vi "Get SMO RC Type.vi"(8 "error in (no error)":errorcluster, 11 "ExampleInstrument in":refnum<class "Instrument.Element2.lvclass">) -> (0 "error out":errorcluster, 2 "Configuration.SMO.RC Type":T1=enum."STM", 3 "ExampleInstrument out":refnum<class "Instrument.Element2.lvclass">)   [LabVIEW 2019, in "Instrument.Element2.lvclass"]
uses:
  Instrument.Element2.lvclass
  <userlib>/LevyLab/Instrument Framework/SMOs/RemoteControl/Typedefs/RC Com Type--enum.ctl
  <userlib>/LevyLab/Instrument Framework/Instrument Types/VSource/Instrument.VSource.lvclass
  <userlib>/LevyLab/Instrument Framework/SMOs/RemoteControl/RemoteControl.lvclass
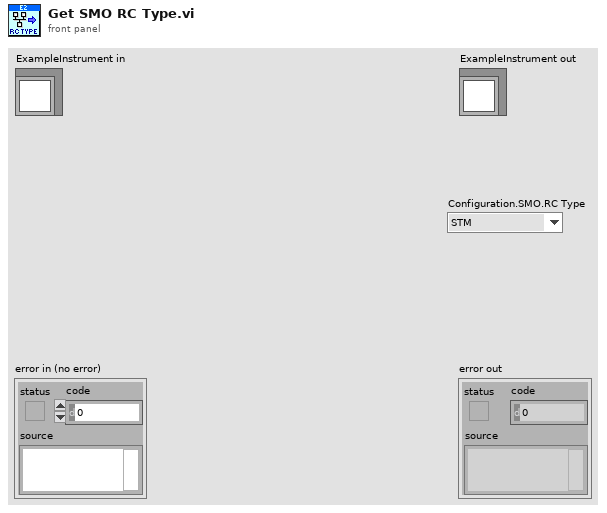
[diagram p1: front panel]
types:
  T1 = typedef "RemoteControl.lvclass/RC Com Type--enum.ctl" = enum16{"RC", "STM", "ZMQ"}
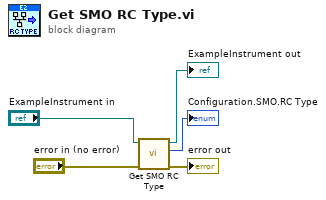
[diagram p0: block diagram]
diagram:
  n1 = call-parent "Get SMO RC Type.vi"("error in (no error)"="error in (no error)", "Instrument in"="ExampleInstrument in") -> ("error out"=→"error out":errorcluster, "RC Type"=→"Configuration.SMO.RC Type":T1, "Instrument out"=→"ExampleInstrument out":refnum<class "Instrument.Element2.lvclass">)  [unwired: 7 in]
